vi "test Inhibit Bus A - RT 2.vi"(8 "error in (no error)":errorcluster, 11 "RT Inhibit Bus A in":refnum<class "RT Inhibit Bus A.lvclass">) -> (0 "error out":errorcluster, 3 "RT Inhibit Bus A out":refnum<class "RT Inhibit Bus A.lvclass">)   [LabVIEW 2016, in "RT Inhibit Bus A.lvclass"]
uses:
  RT Inhibit Bus A.lvclass
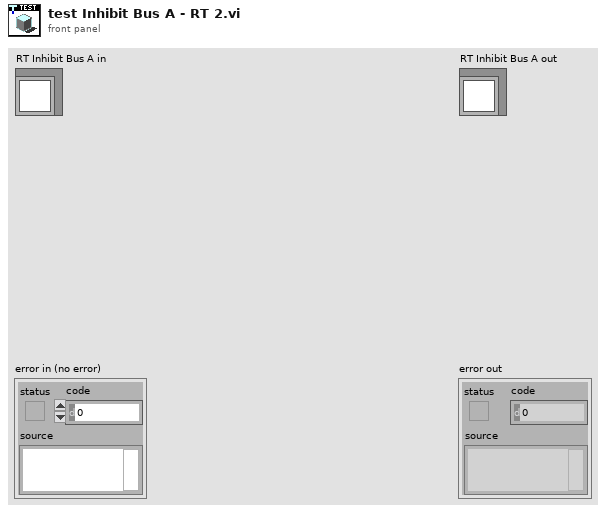
[diagram p1: front panel]
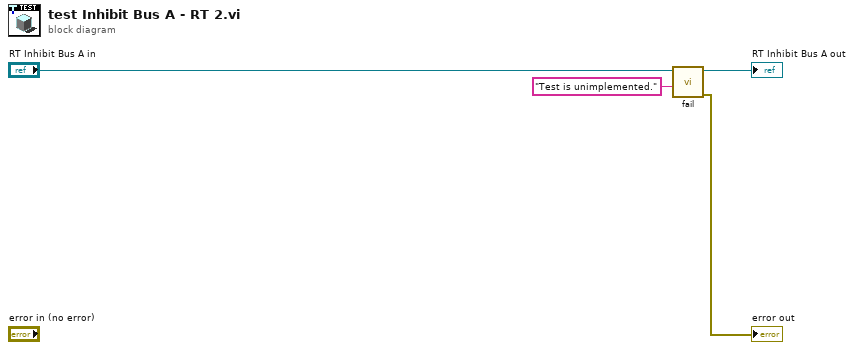
[diagram p0: block diagram]
diagram:
  n1 = call-dynamic "fail.vi"("message (\"\")"="Test is unimplemented." ("message (\"\")"), "TestCase in"="RT Inhibit Bus A in") -> ("error out"=→"error out":errorcluster, "TestCase out"=→"RT Inhibit Bus A out":refnum<class "RT Inhibit Bus A.lvclass">)  [unwired: 8 in]
